vi "serial_read_command.vi"() -> ()   [LabVIEW 2019]
panel:
  out "checksum":u16
  out "data":string
  out "hex integer string":string
  out "length":u8
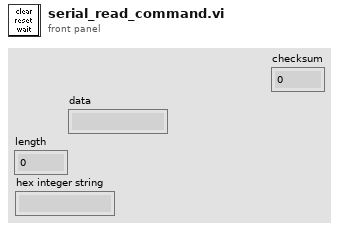
[diagram p1: front panel]
types:
  T1 = enum16{"basic configuration", "test configuration", "converter configuration", "reset", "start", "next cell", "next state"}
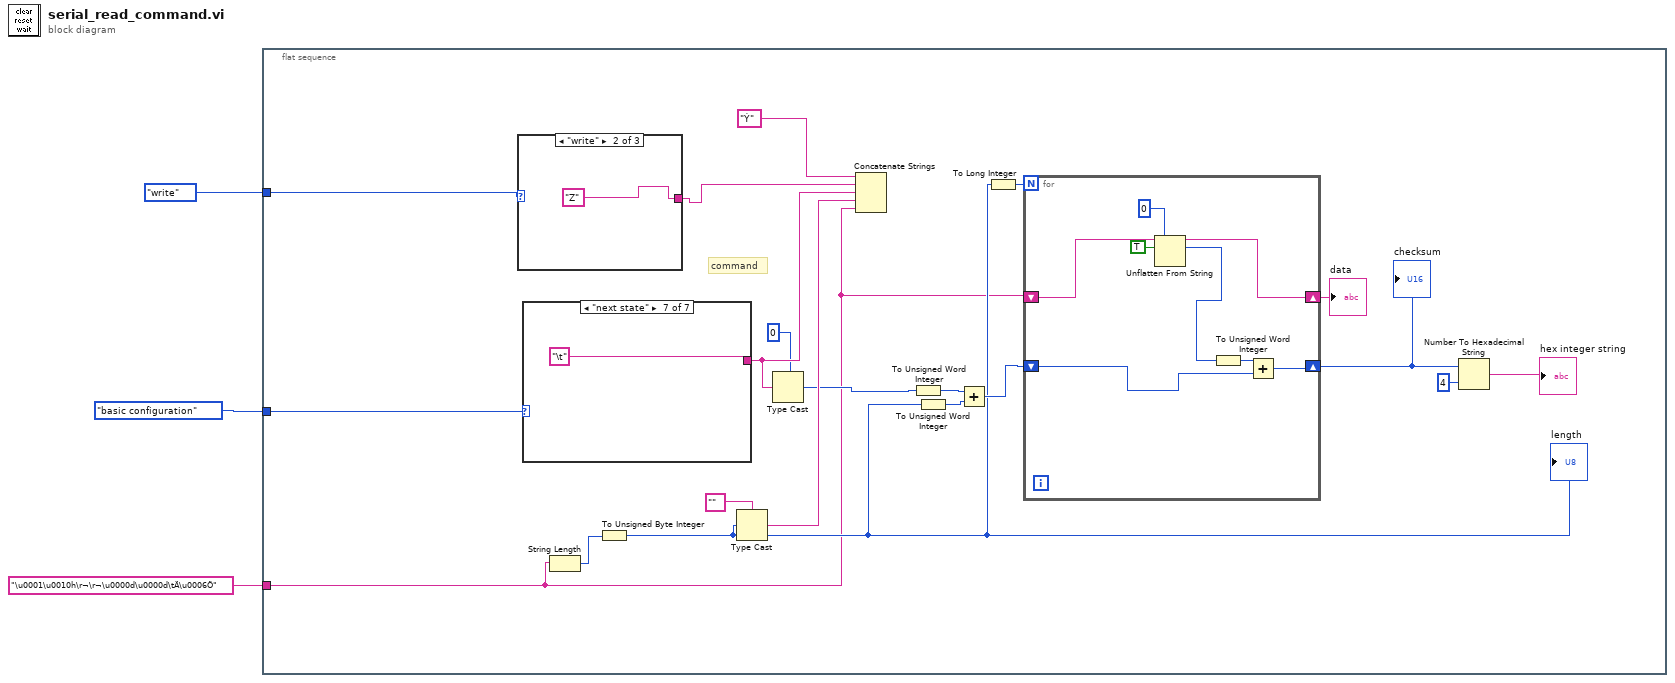
[diagram p0: block diagram]
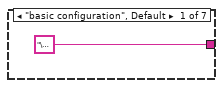
[diagram p2: hidden frame]
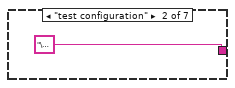
[diagram p3: hidden frame]
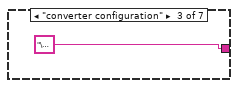
[diagram p4: hidden frame]
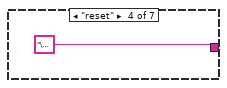
[diagram p5: hidden frame]
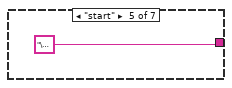
[diagram p6: hidden frame]
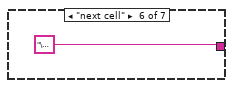
[diagram p7: hidden frame]
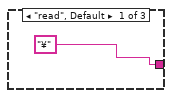
[diagram p8: hidden frame]
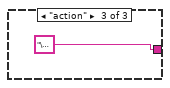
[diagram p9: hidden frame]
diagram:
  n1 = flat-sequence {
    tunnel: enum16{"read", "write", "action"}."write" ("operation") -> [w23]
    tunnel: T1."basic configuration" ("command code") -> [w5]
    tunnel: "\u0001\u0010h\r¬\r¬\u0000d\u0000d\tÄ\u0006Ö" ("data") -> [w4]
    frame #0 {
      # "command"
      n2 = case shown="\"write\"" w23 {
        tunnel: ["¥" "Z" "\u000f"] -> w22
        frame "read", Default {
        }
        frame "write" {
        }
        frame "action" {
        }
      }
      n3 = case shown="\"next state\"" w5 {
        tunnel: ["\u0003" "\u0005" "\u0007" "\u0003" "\u0005" "\u0007" "\t"] -> w18
        frame "basic configuration", Default {
        }
        frame "test configuration" {
        }
        frame "converter configuration" {
        }
        frame "reset" {
        }
        frame "start" {
        }
        frame "next cell" {
        }
        frame "next state" {
        }
      }
      n4 = String Length(string=w4) -> (length=w19:i32)
      n5 = To Unsigned Byte Integer(number=w19) -> (unsigned 8bit integer=w7:u8)
      "length" <- w7
      n6 = Type Cast(type="", x=w7) -> (*(type *) &x=w21:string)
      n7 = Type Cast(type=u8 0, x=w18) -> (*(type *) &x=w10:u8)
      n8 = Concatenate Strings("Ý" ("string"), w22, w18, w21, w4) -> ()  [unwired: 1 out]
      n9 = To Unsigned Word Integer(number=w10) -> (unsigned 16bit integer=w9:u16)
      n10 = To Unsigned Word Integer(number=w7) -> (unsigned 16bit integer=w8:u16)
      n11 = Add(x=w9, y=w8) -> (x+y=w15:u16)
      n12 = To Long Integer(number=w7) -> (32bit integer=w16:i32)
      n13 = for {
        N: w16 -> [_]
        shift-right: [w26] -> w6
        shift-left: w15 -> [w31]
        shift-right: [w27] -> w11
        shift-left: w4 -> [w30]
        n14 = Unflatten From String(type=u8 0, binary string=w30, data includes array or string size? (T)=TRUE) -> (rest of the binary string=w27:string, value=w24:u8)  [unwired: 2 in, 1 out]
        n15 = To Unsigned Word Integer(number=w24) -> (unsigned 16bit integer=w25:u16)
        n16 = Add(x=w25, y=w31) -> (x+y=w26:u16)
      }
      "data" <- w11
      "checksum" <- w6
      n17 = Number To Hexadecimal String(1:i16 4 ("width (-)"), 2:w6) -> (0:→"hex integer string":string)
    }
  }
